vi "talk to RF board (FPGA).vi"() -> ()   [LabVIEW 2009]
doc: "UHR-Fleezers Instrument Control Code (fpga)"
uses:
  <vilib>/Platform/TimedLoop/XDataNode/XDataNode.xnode
  <vilib>/Platform/TimedLoop/XDataNode/loadlvalarms.vi
  <vilib>/Platform/TimedLoop/XDataNode/timing_clust.ctl
  <vilib>/Platform/TimedLoop/XDataNode/nitl_modes.ctl
  <vilib>/Platform/TimedLoop/XDataNode/wakeup.ctl
  <vilib>/eio/EIOMethodNode/EIOMethodNode.xnode
  <vilib>/rvi/eio/nirviEIOMethodImplementation/nirviEIOMethodImplementation.xnode
  <vilib>/rvi/eio/common/nirviEmuTemplateMethod_noerrors.vi
  <vilib>/rvi/eio/common/nirviEmuClasses.ctl
  <vilib>/eio/EIONode/EIONode.xnode
  <vilib>/rvi/eio/nirviEIOImplementation/nirviEIOImplementation.xnode
  <vilib>/Platform/TimedLoop/XDataNode/XDNodeRunTimeDep.lvlib
panel:
  in  "Tab Control":T1(tab)
  in  "Tab Control 2":T2(tab)
  in  "OSK Bd 1":bool
  in  "Reset Bd 1":bool
  in  "RD":bool
  in  "PMODE":bool
  in  "OSK Bd 2":bool
  in  "Reset Bd 2":bool
  in  "Direct RF Box \nCommunication":bool
  in  "Data BD 2":u8 format="%08b"
  in  "Data BD 1":u8 format="%08b"
  in  "Address":u8 format="%02x"
  in  "Update Data":bool
  # "Only one of these can be on\nat a time:"
  # "Raster Scan AOD"
  # "1 (X)"
  # "2 (Y)"
  # "IR Intensity Feedback (RF BD 1)"
  # "AO1 (Y)"
  # "2D"
  # "1D"
  # "AO2 (X)"
  # "APD AO for aligning"
  # "Detection Loop"
  # "Green fluorescent laser digital gate interlacing loop"
  # "0 Forced ON\n1 Forced OFF\n2 Interlacing"
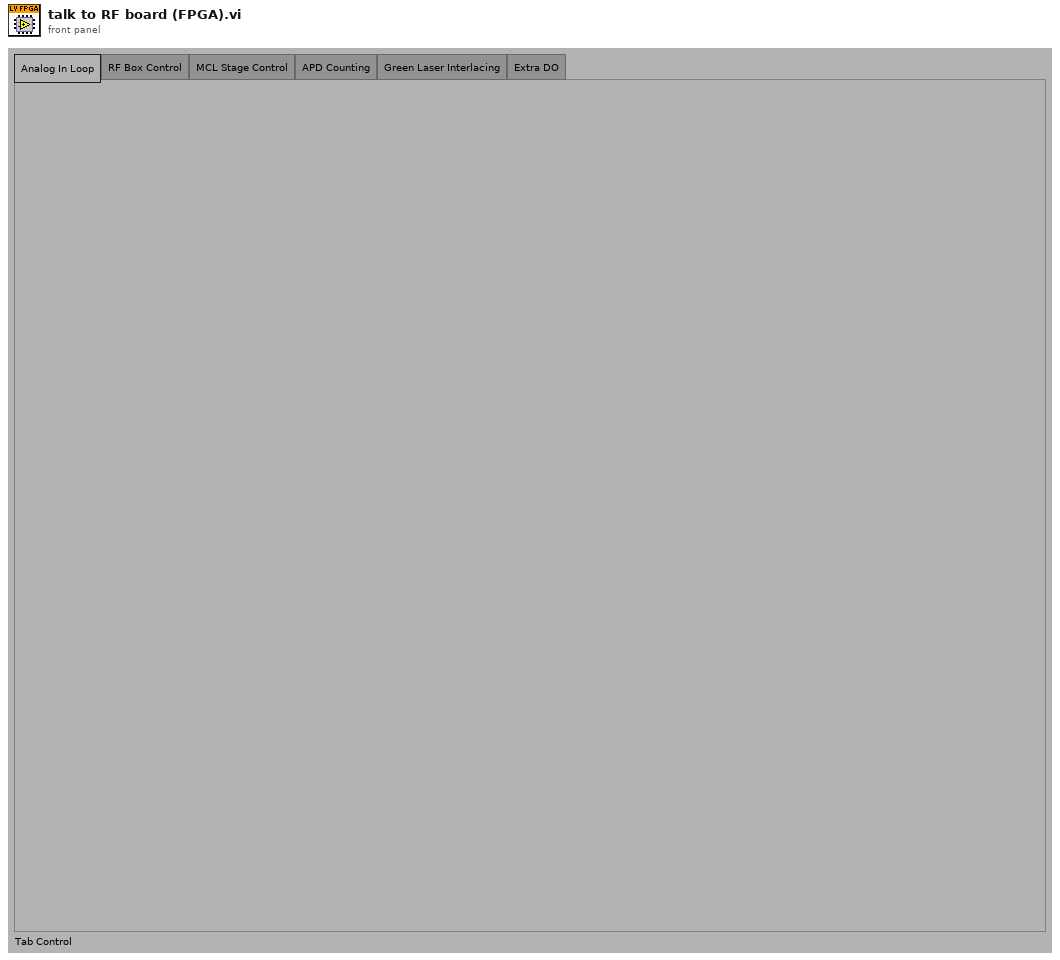
[diagram p1: front panel]
types:
  T1 = enum32{"Analog In Loop", "RF Box Control", "MCL Stage Control", "APD Counting", "Green Laser Interlacing", "Extra DO"}
  T2 = enum32{"Controls", "Interlacing Frequency and Amplitude Values"}
  T3 = typedef "nirviEmuClasses.ctl" = enum16{"IO Read", "IO Write", "Method", "Property Read", "Property Write"}
  T4 = typedef "XDNodeRunTimeDep.lvlib/timing_clust.ctl" = cluster{"Expected End [f-1]":u64, "Actual End [f-1]":u64, "Finished Late? [f-1]":bool, "Expected End [i-1]":u64, "Actual End [i-1]":u64, "Finished Late? [i-1]":bool, "Expected Start [i]":u64, "Actual Start [i]":u64, "Expected Start [f]":u64, "Actual Start [f]":u64, "Source Name":string, "Structure Name":string, "Period":i64, "Deadline":i64, "Offset":i64, "Start":i64, "Priority":i32, "Timeout":i32, "Mode":T5, "Wakeup Reason":T6, "Error":errorcluster, "Source Type":string, "Secondary Source Type":string, "Global End Time":u64, "Global Start Time":u64, "Frame Duration":u64, "Iteration Duration":u64, "Assigned CPU":i32, "I/O Scan Engine Mode":u32}
  T5 = typedef "XDNodeRunTimeDep.lvlib/nitl_modes.ctl" = enum32{"No Change", "Process missed periods, maintain original phase", "Discard missed periods, maintain original phase", "Process missed periods, ignore original phase", "Discard missed periods, ignore original phase"}
  T6 = typedef "XDNodeRunTimeDep.lvlib/wakeup.ctl" = enum32{"Normal", "Aborted", "Asynchronous wakeup", "Timing source error", "Timed loop error", "Timeout"}
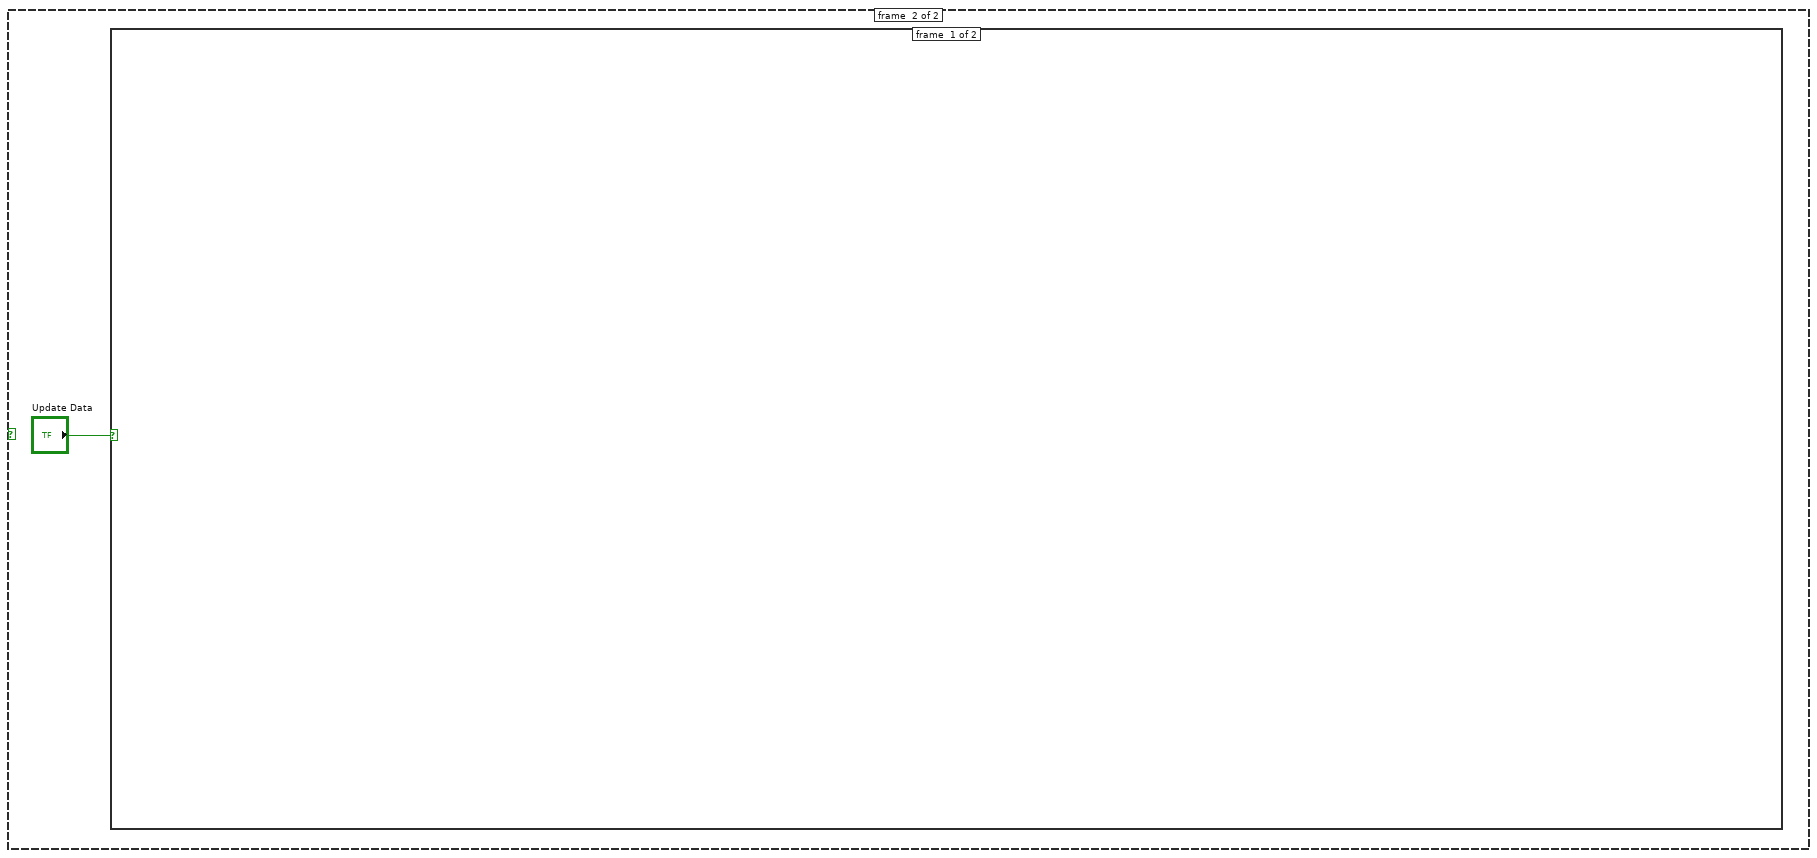
[diagram p2: hidden frame]
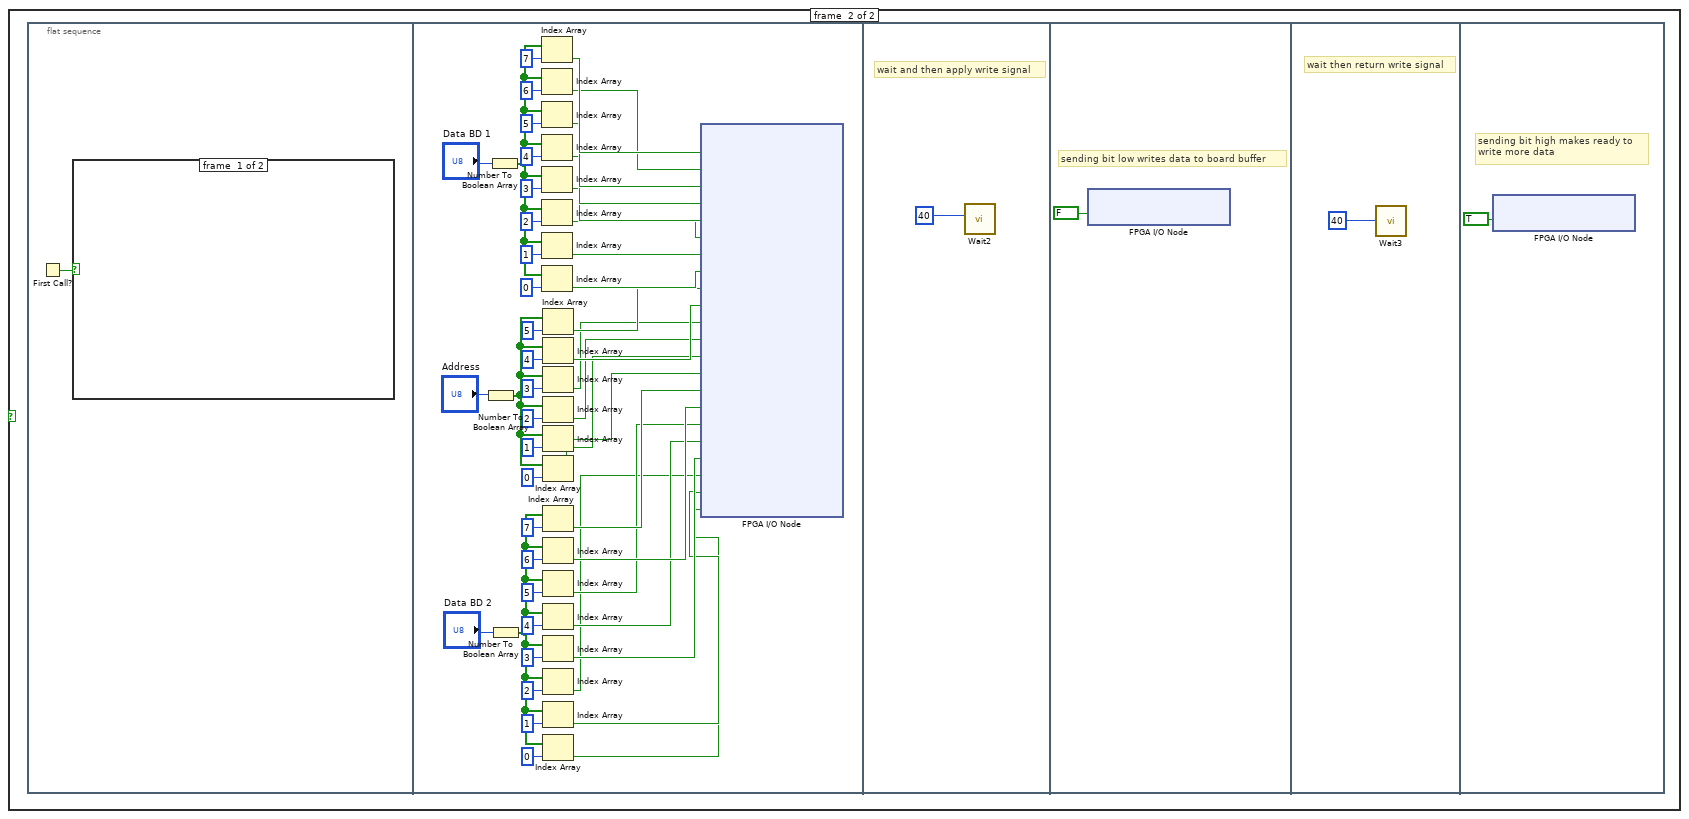
[diagram p3: hidden frame]
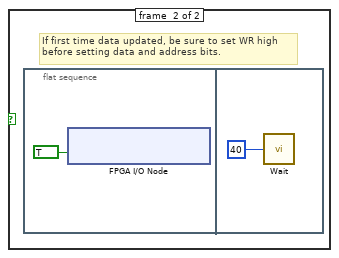
[diagram p4: hidden frame]
diagram:
  (unwired) FALSE
  (unwired) FALSE
  # "timing array current index"
  # "timing array"
  # "timing counter (phase adjusted here)"
  # "late counter"
  n1 = flat-sequence "FPGA initialization to do before running any of the loops" {
    tunnel: [u32 0 ("DIO count 3 (ticks)")] -> w1
    frame #0 {
      # "This pin controls udclk on the RF boards.\nWhen initially configuring the boards, this pin needs to be\nconfigured as a high impedance input.  Later it will be switched\nto an output."
      # "Initial setting of DIO data and \naddress to low (before reset).  \nThis needs to happen before the other\ncontrol method loops execute."
      n2 = xnode "FPGA I/O Node"("Connector1/DIO0"=FALSE, "Connector1/DIO1"=FALSE, "Connector1/DIO2"=FALSE, "Connector1/DIO3"=FALSE, "Connector1/DIO4"=FALSE, "Connector1/DIO5"=FALSE, "Connector1/DIO6"=FALSE, "Connector1/DIO7"=FALSE, "Connector1/DIO8"=FALSE, "Connector1/DIO9"=FALSE, "Connector1/DIO10"=FALSE, "Connector1/DIO11"=FALSE, "Connector1/DIO12"=FALSE, "Connector1/DIO13"=FALSE, "Connector1/DIO15"=FALSE, "Connector1/DIO20"=FALSE, "Connector1/DIO21"=FALSE, "Connector1/DIO22"=FALSE, "Connector1/DIO23"=FALSE, "Connector1/DIO24"=FALSE, "Connector1/DIO25"=FALSE, "Connector1/DIO26"=FALSE, "Connector1/DIO27"=FALSE, "Connector1/DIO14"=FALSE) -> ()  [unwired: 24 in, 24 out]
      n3 = xnode "FPGA I/O Method Node"("Enable"=FALSE) -> ()  [unwired: 1 in, 1 out]
    }
  }
  n4 = while "RF box board direct communication loop" {
    tunnel: w1 -> [_]
    stop <- FALSE stop-if-true
    n5 = case "Whether to use direct communication method (only use one method at a time)" shown="True" "Direct RF Box \nCommunication" {
      frame #0 {
      }
      frame #1 {
        n6 = case shown="True" "Update Data" {
          frame #0 {
          }
          frame #1 {
            n7 = flat-sequence {
              frame #0 {
                n8 = First Call?() -> (First Call?: T/F=w356:bool)
                n9 = case shown="True" w356 {
                  frame #0 {
                  }
                  frame #1 {
                    # "If first time data updated, be sure to set WR high\nbefore setting data and address bits."
                    n10 = flat-sequence {
                      frame #0 {
                        n11 = xnode "FPGA I/O Node"("Connector1/DIO15"=TRUE) -> ()  [unwired: 1 in, 1 out]
                      }
                      frame #1 {
                        n12 = call "Wait"("Count(Ticks)"=u8 40 ("DO Delay 3 (Ticks)")) -> ()  [unwired: 1 out]
                      }
                    }
                  }
                }
              }
              frame #1 {
                n13 = Number To Boolean Array(number="Address") -> (Boolean array=w418:bool[])
                n14 = Number To Boolean Array(number="Data BD 1") -> (Boolean array=w419:bool[])
                n15 = Number To Boolean Array(number="Data BD 2") -> (Boolean array=w388:bool[])
                n16 = Index Array(array=w419, index=7) -> (element=w403:bool)
                n17 = Index Array(array=w419, index=6) -> (element=w402:bool)
                n18 = Index Array(array=w419, index=5) -> (element=w401:bool)
                n19 = Index Array(array=w419, index=4) -> (element=w400:bool)
                n20 = Index Array(array=w419, index=3) -> (element=w399:bool)
                n21 = Index Array(array=w419, index=2) -> (element=w398:bool)
                n22 = Index Array(array=w419, index=1) -> (element=w397:bool)
                n23 = Index Array(array=w419, index=0) -> (element=w396:bool)
                n24 = Index Array(array=w418, index=5) -> (element=w395:bool)
                n25 = Index Array(array=w418, index=4) -> (element=w394:bool)
                n26 = Index Array(array=w418, index=3) -> (element=w393:bool)
                n27 = Index Array(array=w418, index=2) -> (element=w392:bool)
                n28 = Index Array(array=w418, index=1) -> (element=w391:bool)
                n29 = Index Array(array=w418, index=0) -> (element=w390:bool)
                n30 = Index Array(array=w388, index=7) -> (element=w379:bool)
                n31 = Index Array(array=w388, index=6) -> (element=w378:bool)
                n32 = Index Array(array=w388, index=5) -> (element=w377:bool)
                n33 = Index Array(array=w388, index=4) -> (element=w376:bool)
                n34 = Index Array(array=w388, index=3) -> (element=w375:bool)
                n35 = Index Array(array=w388, index=2) -> (element=w374:bool)
                n36 = Index Array(array=w388, index=1) -> (element=w373:bool)
                n37 = Index Array(array=w388, index=0) -> (element=w372:bool)
                n38 = xnode "FPGA I/O Node"("Connector1/DIO0"=w403, "Connector1/DIO1"=w402, "Connector1/DIO2"=w401, "Connector1/DIO3"=w400, "Connector1/DIO4"=w399, "Connector1/DIO5"=w398, "Connector1/DIO6"=w397, "Connector1/DIO7"=w396, "Connector1/DIO8"=w395, "Connector1/DIO9"=w394, "Connector1/DIO10"=w393, "Connector1/DIO11"=w392, "Connector1/DIO12"=w391, "Connector1/DIO13"=w390, "Connector1/DIO20"=w379, "Connector1/DIO21"=w378, "Connector1/DIO22"=w377, "Connector1/DIO23"=w376, "Connector1/DIO24"=w375, "Connector1/DIO25"=w374, "Connector1/DIO26"=w373, "Connector1/DIO27"=w372) -> ()  [unwired: 22 in, 22 out]
              }
              frame #2 {
                # "wait and then apply write signal"
                n39 = call "Wait2"("Count(Ticks)"=u8 40 ("DO Delay 1 (Ticks)")) -> ()  [unwired: 1 out]
              }
              frame #3 {
                # "sending bit low writes data to board buffer"
                n40 = xnode "FPGA I/O Node"("Connector1/DIO15"=FALSE) -> ()  [unwired: 1 in, 1 out]
              }
              frame #4 {
                # "wait then return write signal"
                n41 = call "Wait3"("Count(Ticks)"=u8 40 ("DO Delay 2 (Ticks)")) -> ()  [unwired: 1 out]
              }
              frame #5 {
                # "sending bit high makes ready to\nwrite more data"
                n42 = xnode "FPGA I/O Node"("Connector1/DIO15"=TRUE) -> ()  [unwired: 1 in, 1 out]
              }
            }
          }
        }
      }
    }
  }
  n43 = node-c288() -> (w3:T4)  [unwired: 1 in]
  n44 = timed-loop "RF box board DIO control: control bits" {
    timing: w3 -> [_]
    timing-out: [_] -> w2
    tunnel: [w738] -> _
    tunnel: w1 -> [w738]
    stop <- FALSE stop-if-true
    n45 = xnode "FPGA I/O Node"("Connector1/DIO16"="RD", "Connector1/DIO17"="PMODE", "Connector1/DIO18"="OSK Bd 1", "Connector1/DIO19"="Reset Bd 1", "Connector1/DIO28"="OSK Bd 2", "Connector1/DIO29"="Reset Bd 2") -> ()  [unwired: 6 in, 6 out]
  }
  n46 = node-c288(w2) -> ()
